vi "string 2 double.vi"(2 "string":string) -> (16 "number":dbl format="%#_15f", 17 "scanned string":string, 18 "length":u8, 19 "precision":u8)   [LabVIEW 2014, in "PTUtils.lvlib"]
uses:
  PTUtils.lvlib
  <vilib>/regexp/Match Regular Expression.xnode
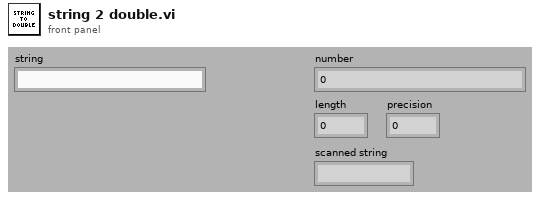
[diagram p1: front panel]
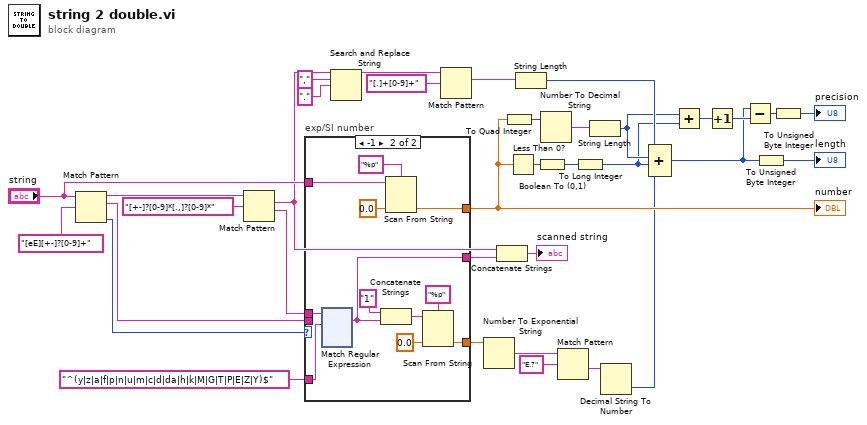
[diagram p0: block diagram]
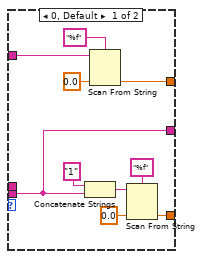
[diagram p2: hidden frame]
diagram:
  n1 = Match Pattern(string="string", regular expression="[eE][+-]?[0-9]+") -> (before substring=w32:string, match substring=w34:string, offset past match=w18:i32)  [unwired: 1 in, 1 out]
  n2 = Match Pattern(string=w32, regular expression="[+-]?[0-9]*[.,]?[0-9]*") -> (match substring=w15:string, after substring=w31:string)  [unwired: 1 in, 2 out]
  n3 = case "exp/SI number" shown="-1" w18 {
    tunnel: w34 -> [w36 _]
    tunnel: w31 -> [_ w54]
    tunnel: [w42 w53] -> w20
    tunnel: "^(y|z|a|f|p|n|u|m|c|d|da|h|k|M|G|T|P|E|Z|Y)$" -> [_ w51]
    tunnel: "string" -> [w39 w49]
    tunnel: [w37 w47] -> w12
    tunnel: [w36 w46] -> w16
    frame 0, Default {
      n4 = Concatenate Strings("1", w36) -> (w43:string)
      n5 = Scan From String(format string="%f", input string=w39, default 1=0.0 ("default value 1")) -> (output 1=w37:dbl)  [unwired: 2 in, 3 out]
      n6 = Scan From String(format string="%f", input string=w43, default 1=0.0 ("default value 1")) -> (output 1=w42:dbl)  [unwired: 2 in, 3 out]
    }
    frame -1 {
      n7 = xnode "Match Regular Expression"("input string"=w54, "regular expression"=w51) -> ("whole match"=w46:string)  [unwired: 4 in, 4 out]
      n8 = Concatenate Strings("1", w46) -> (w56:string)
      n9 = Scan From String(format string="%p", input string=w49, default 1=0.0 ("default value 1")) -> (output 1=w47:dbl)  [unwired: 2 in, 3 out]
      n10 = Scan From String(format string="%p", input string=w56, default 1=0.0 ("default value 1")) -> (output 1=w53:dbl)  [unwired: 2 in, 3 out]
    }
  }
  "number" <- w12
  n11 = Search and Replace String(input string=w15, search string=",", replace string=".") -> (result string=w26:string)  [unwired: 5 in, 3 out]
  n12 = Match Pattern(string=w26, regular expression="[.]+[0-9]+") -> (match substring=w19:string)  [unwired: 1 in, 3 out]
  n13 = Number To Exponential String(number=w20) -> (E-format string=w24:string)  [unwired: 3 in]
  n14 = Concatenate Strings(w15, w16) -> (→"scanned string":string)
  n15 = To Quad Integer(1:w12) -> (0:w22:i64)
  n16 = Less Than 0?(x=w12) -> (x < 0?=w9:bool)
  n17 = String Length(string=w19) -> (length=w14:i32)
  n18 = Boolean To (0,1)(Boolean=w9) -> (0, 1=w7:i16)
  n19 = Number To Decimal String(number=w22) -> (decimal integer string=w21:string)  [unwired: 1 in]
  n20 = Match Pattern(string=w24, regular expression="E.?") -> (after substring=w23:string)  [unwired: 1 in, 3 out]
  n21 = To Long Integer(number=w7) -> (32bit integer=w6:i32)
  n22 = String Length(string=w21) -> (length=w8:i32)
  n23 = Decimal String To Number(string=w23) -> (number=w10:i32)  [unwired: 2 in, 1 out]
  n24 = Compound Arithmetic op=ADD(w14, w8, w6, w10) -> (w3:i32)
  n25 = Add(x=w8, y=w6) -> (x+y=w5:i32)
  n26 = Increment(x=w5) -> (x+1=w4:i32)
  n27 = Subtract(x=w3, y=w4) -> (x-y=w2:i32)
  n28 = To Unsigned Byte Integer(number=w3) -> (unsigned 8bit integer=→"length":u8)
  n29 = To Unsigned Byte Integer(number=w2) -> (unsigned 8bit integer=→"precision":u8)
